vi "PORT IO Read__ogtk.vi"   [LabVIEW 2014]
doc: "This function reads data from the specified IO port. If you set fast to True, and are running under Windows NT/2000/XP/2003 you must have enabled the according IO port with a call to \"PORT IO Enable Range.vi\" to avoid a General Protection Fault error."
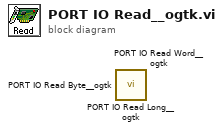
[diagram p0: block diagram]
diagram:
  n1 = call <userlib>:"PORT IO Read Long__ogtk.vi"() -> ()  [unwired: 6 in, 2 out]
  n2 = call <userlib>:"PORT IO Read Word__ogtk.vi"() -> ()  [unwired: 6 in, 2 out]
  n3 = call <userlib>:"PORT IO Read Byte__ogtk.vi"() -> ()  [unwired: 6 in, 2 out]
